vi "ThickLine(SubVI).vi"(7 "Color":u32=16775680, 8 "error in (no error)":errorcluster, 9 "End Point Coordinates":cluster{"X (m)":sgl, "Y (m)":sgl}={"X (m)"=-1.8998767e-07, "Y (m)"=-2.066301e-07}, 10 "End Point Coordinates 2":cluster{"X (m)":sgl, "Y (m)":sgl}={"X (m)"=-1.817262e-07, "Y (m)"=-2.0885543e-07}, 11 "Application in":refnum<vi>) -> (0 "error out":errorcluster, 3 "Application out":refnum<vi>)   [LabVIEW 2014]
uses:
  <userlib>/Nanonis Prog Interface V5/Nanonis Prog Interface.lvlib
panel:
  in  "spread":sgl=0.5
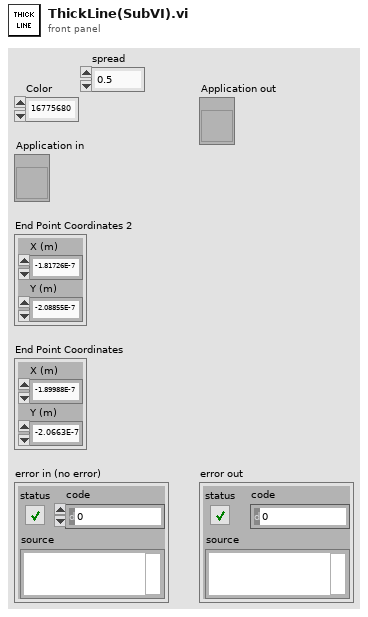
[diagram p1: front panel]
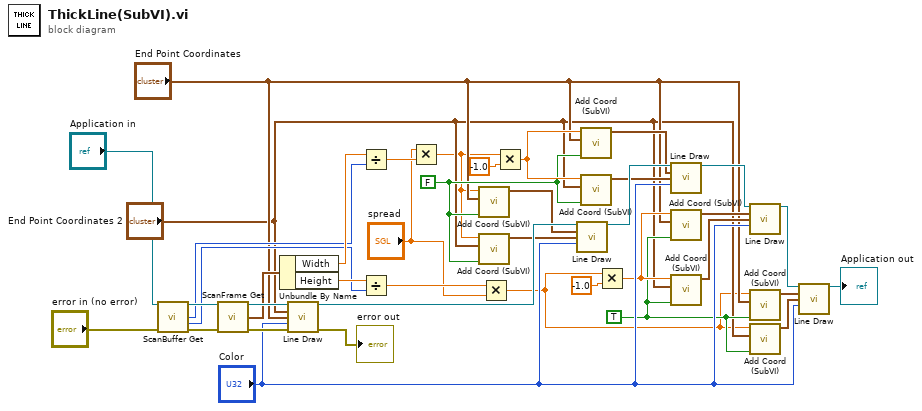
[diagram p0: block diagram]
diagram:
  w10 = TRUE ("X")
  w17 = FALSE ("X")
  n1 = call <userlib>:"ScanBuffer Get.vi"("Application ref in"="Application in", "error in (no error)"="error in (no error)") -> ("Application ref out"=w36:refnum<vi>, "Pixels/line"=w29:i32, "Lines"=w28:i32, "error out"=w34:errorcluster)  [unwired: 9 in, 1 out]
  n2 = call <userlib>:"ScanFrame Get.vi"("Application ref in"=w36, "error in (no error)"=w34) -> ("Application ref out"=w38:refnum<vi>, "Size (m)"=w32:cluster{"Width":sgl, "Height":sgl}, "error out"=w33:errorcluster)  [unwired: 9 in, 2 out]
  n3 = Unbundle By Name(w32) -> ("Width"=w31:sgl, "Height"=w30:sgl)
  n4 = call <userlib>:"Line Draw.vi"("Application ref in"=w38, "Start Point Coordinates"="End Point Coordinates 2", "End Point Coordinates"="End Point Coordinates", "Color"="Color", "error in (no error)"=w33) -> ("Application ref out"=w27:refnum<vi>, "error out"=→"error out":errorcluster)  [unwired: 9 in]
  n5 = Divide(x=w31, y=w29) -> (x/y=w20:sgl)
  n6 = Divide(x=w30, y=w28) -> (x/y=w11:sgl)
  n7 = Multiply(x="spread", y=w20) -> (x*y=w3:sgl)
  n8 = call "Add Coord (SubVI).vi"("X"=w17, "End Point Coordinates in"="End Point Coordinates", "Numeric"=w3) -> ("End Point Coordinates out"=w22:cluster{"X (m)":sgl, "Y (m)":sgl})  [unwired: 8 in]
  n9 = call "Add Coord (SubVI).vi"("X"=w17, "End Point Coordinates in"="End Point Coordinates 2", "Numeric"=w3) -> ("End Point Coordinates out"=w21:cluster{"X (m)":sgl, "Y (m)":sgl})  [unwired: 8 in]
  n10 = Multiply(x=w11, y="spread") -> (x*y=w2:sgl)
  n11 = Multiply(x=w3, y=sgl -1.0) -> (x*y=w18:sgl)
  n12 = call <userlib>:"Line Draw.vi"("Application ref in"=w27, "Start Point Coordinates"=w22, "End Point Coordinates"=w21, "Color"="Color") -> ("Application ref out"=w26:refnum<vi>)  [unwired: 10 in, 1 out]
  n13 = call "Add Coord (SubVI).vi"("X"=w17, "End Point Coordinates in"="End Point Coordinates", "Numeric"=w18) -> ("End Point Coordinates out"=w16:cluster{"X (m)":sgl, "Y (m)":sgl})  [unwired: 8 in]
  n14 = call "Add Coord (SubVI).vi"("X"=w17, "End Point Coordinates in"="End Point Coordinates 2", "Numeric"=w18) -> ("End Point Coordinates out"=w15:cluster{"X (m)":sgl, "Y (m)":sgl})  [unwired: 8 in]
  n15 = Multiply(x=w2, y=sgl -1.0) -> (x*y=w12:sgl)
  n16 = call <userlib>:"Line Draw.vi"("Application ref in"=w26, "Start Point Coordinates"=w16, "End Point Coordinates"=w15, "Color"="Color") -> ("Application ref out"=w24:refnum<vi>)  [unwired: 10 in, 1 out]
  n17 = call "Add Coord (SubVI).vi"("X"=w10, "End Point Coordinates in"="End Point Coordinates", "Numeric"=w12) -> ("End Point Coordinates out"=w9:cluster{"X (m)":sgl, "Y (m)":sgl})  [unwired: 8 in]
  n18 = call "Add Coord (SubVI).vi"("X"=w10, "End Point Coordinates in"="End Point Coordinates 2", "Numeric"=w12) -> ("End Point Coordinates out"=w8:cluster{"X (m)":sgl, "Y (m)":sgl})  [unwired: 8 in]
  n19 = call <userlib>:"Line Draw.vi"("Application ref in"=w24, "Start Point Coordinates"=w9, "End Point Coordinates"=w8, "Color"="Color") -> ("Application ref out"=w25:refnum<vi>)  [unwired: 10 in, 1 out]
  n20 = call "Add Coord (SubVI).vi"("X"=w10, "End Point Coordinates in"="End Point Coordinates", "Numeric"=w2) -> ("End Point Coordinates out"=w7:cluster{"X (m)":sgl, "Y (m)":sgl})  [unwired: 8 in]
  n21 = call "Add Coord (SubVI).vi"("X"=w10, "End Point Coordinates in"="End Point Coordinates 2", "Numeric"=w2) -> ("End Point Coordinates out"=w6:cluster{"X (m)":sgl, "Y (m)":sgl})  [unwired: 8 in]
  n22 = call <userlib>:"Line Draw.vi"("Application ref in"=w25, "Start Point Coordinates"=w7, "End Point Coordinates"=w6, "Color"="Color") -> ("Application ref out"=→"Application out":refnum<vi>)  [unwired: 10 in, 1 out]
